vi "OE2012&OE2022_Configure Trig.vi"(6 "Trig Mode":u8(ring) items=["Ext_Rissing_Edge", "Ext_Falling_Edge", "Ext_Bilateral_Edge", "Ext_High_Level", "Ext_Low_Level"], 7 "Trig Source":u8(ring) items=["Internal", "Aux-in1", "Aux-in2"], 8 "Error in (no error)":errorcluster caption="error out（no error）", 9 "Remote Mode":u16(ring)=1 items=["USB", "RS232", "GPIB", "Ethernet"], 10 "Connection ID in":refnum<k5>, 11 "VISA resource name":refnum<visa-resource-name>) -> (0 "Error out":errorcluster caption="error out", 1 "Output String":string, 2 "Connection ID out":refnum<k5>, 3 "VISA resource  out":refnum<visa-resource-name>)   [LabVIEW 2011]
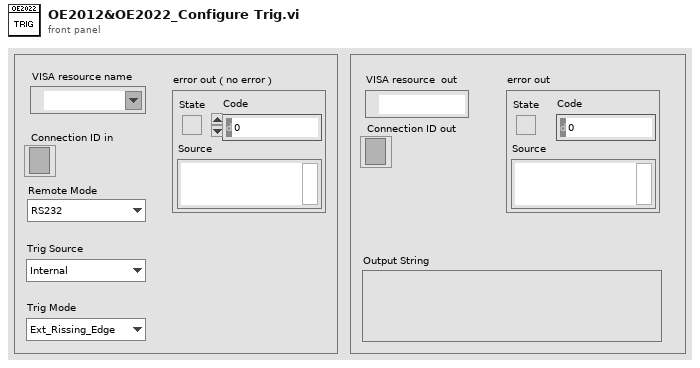
[diagram p1: front panel]
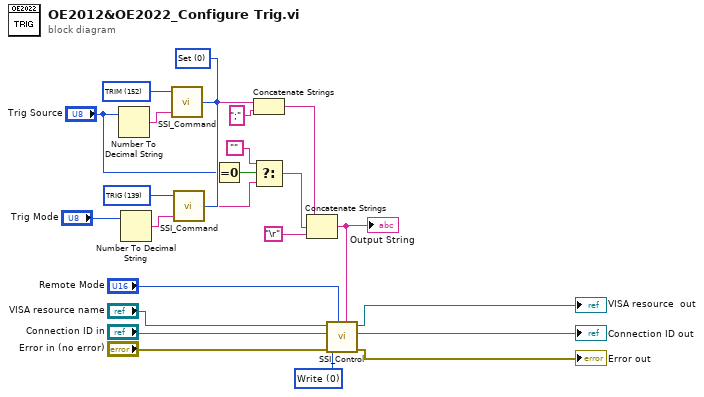
[diagram p0: block diagram]
diagram:
  w10 = u16 152 items=["ISRC", "IGND", "ICPL", "ILIN", "PHAS", "FMOD", "RSLP", "FREQ", "SWPT", "SLLM", "SULM", "SSLL", "SSLG", "STLM", "SWRM", "IRNG", "SENS", "RMOD", "OFLT", "OFSL", "SYNC", "DMOD", "HARM", "DARB", "SWVT", "SLVL", "SVLL", "SVUL", "SVSL", "SVSG", "SVTM", "SVRM", "RALL", "SNAP", "OUTP", "OAUX", "COUT", "CAUX", "COFP", "CEXP", "FPOP", "OEXP", "*IDN", "*RST", "OVLD", "INOV", "GNOV", "*PLL", "SSET", "RSET", "AGAN", "APHS", "ARSV", "ASCL", "EQCD", "EQCS", "SPED", "SRAT", "SLEN", "SSLE", "STRG", "SPRM", "STRD", "PAUS", "REST", "SPTS", "TRCA", "TEMP", "RSTU", "INHZ", "DEQU", "SADD", "ARNG", "CSPE", "ISRCD", "IGNDD", "ICPLD", "ILIND", "PHASD", "FMODD", "RSLPD", "FREQD", "SWPTD", "SLLMD", "SULMD", "SSLLD", "SSLGD", "STLMD", "SWRMD", "SENSD", "RMODD", "OFLTD", "OFSLD", "SYNCD", "HARMD", "EQCDD", "EQCSD", "SNAPD", "OUTPD", "SWVTD", "SLVLD", "SVLLD", "SVULD", "SVSLD", "SVSGD", "SVTMD", "SVRMD", "SVDCD", "ARSVD", "AGAND", "APHSD", "ASCLD", "FPOPD", "CAUXD", "OEXPD", "SPEDD", "SRATD", "SLEND", "SSLED", "STRGD", "SPRMD", "STRDD", "PAUSD", "RESTD", "SPTSD", "TRCAD", "*IDND", "*RSTD", "INOVD", "GNOVD", "*PLLD", "SSETD", "RSETD", "RALLD", "NIPA", "NSMA", "NGWA", "NMAC", "NMOD", "TRIG", "TRCB", "INHZD", "ISAMD", "IRAGD", "RRAGD", "SOFFD", "DMODD", "COUTD", "COFPD", "CEXPD", "ARNGD", "OAUXD", "TRIM"] ("Command Type")
  w14 = u16 0 items=["Write", "Read"] ("Control")
  w20 = u16 139 items=["ISRC", "IGND", "ICPL", "ILIN", "PHAS", "FMOD", "RSLP", "FREQ", "SWPT", "SLLM", "SULM", "SSLL", "SSLG", "STLM", "SWRM", "IRNG", "SENS", "RMOD", "OFLT", "OFSL", "SYNC", "DMOD", "HARM", "DARB", "SWVT", "SLVL", "SVLL", "SVUL", "SVSL", "SVSG", "SVTM", "SVRM", "RALL", "SNAP", "OUTP", "OAUX", "COUT", "CAUX", "COFP", "CEXP", "FPOP", "OEXP", "*IDN", "*RST", "OVLD", "INOV", "GNOV", "*PLL", "SSET", "RSET", "AGAN", "APHS", "ARSV", "ASCL", "EQCD", "EQCS", "SPED", "SRAT", "SLEN", "SSLE", "STRG", "SPRM", "STRD", "PAUS", "RSET", "SPTS", "TRCA", "TEMP", "RSTU", "INHZ", "DEQU", "SADD", "ARNG", "CSPE", "ISRCD", "IGNDD", "ICPLD", "ILIND", "PHASD", "FMODD", "RSLPD", "FREQD", "SWPTD", "SLLMD", "SULMD", "SSLLD", "SSLGD", "STLMD", "SWRMD", "SENSD", "RMODD", "OFLTD", "OFSLD", "SYNCD", "HARMD", "EQCDD", "EQCSD", "SNAPD", "OUTPD", "SWVTD", "SLVLD", "SVLLD", "SVULD", "SVSLD", "SVSGD", "SVTMD", "SVRMD", "SVDCD", "ARSVD", "AGAND", "APHSD", "ASCLD", "FPOPD", "CAUXD", "OEXPD", "SPEDD", "SRATD", "SLEND", "SSLED", "STRGD", "SPRMD", "STRDD", "PAUSD", "RESTD", "SPTSD", "TRCAD", "*IDND", "*RSTD", "INOVD", "GNOVD", "*PLLD", "SSETD", "RSETD", "RALLD", "NIPA", "NSMA", "NGWA", "NMAC", "NMOD", "TRIG"] ("Command Type")
  w9 = u16 0 items=["Set", "Query"] ("Opera")
  n1 = Number To Decimal String(number="Trig Source") -> (decimal integer string=w11:string)  [unwired: 1 in]
  n2 = Number To Decimal String(number="Trig Mode") -> (decimal integer string=w19:string)  [unwired: 1 in]
  n3 = call "SSI_Command.vi"("Opera"=w9, "Paramter"=w11, "Command Type"=w10) -> ("Output string"=w4:string)  [unwired: 1 in]
  n4 = call "SSI_Command.vi"("Opera"=w9, "Paramter"=w19, "Command Type"=w20) -> ("Output string"=w6:string)  [unwired: 1 in]
  n5 = Equal To 0?(x="Trig Source") -> (x = 0?=w8:bool)
  n6 = Concatenate Strings(w4, ";" ("字符串")) -> (w2:string)
  n7 = Select(t="", s=w8, f=w6) -> (s? t:f=w1:string)
  n8 = Concatenate Strings(w2, w1, "\r") -> (w12:string)
  "Output String" <- w12
  n9 = call "SSI_Control.vi"("Write Buffer"=w12, "Remote Mode"="Remote Mode", "Error in (no error)"="Error in (no error)", "Control"=w14, "Connection ID in"="Connection ID in", "VISA resource name"="VISA resource name") -> ("Error out"=→"Error out":errorcluster, "Connection ID out"=→"Connection ID out":refnum<k5>, "VISA resource  out"=→"VISA resource  out":refnum<visa-resource-name>)  [unwired: 2 in, 1 out]
